vi "CRYMR Min Margin.vi"(3 "Lower X":dbl format="%.2f", 4 "Lower Margin":dbl format="%.2p", 5 "Upper X":dbl format="%.2f", 6 "Upper Margin":dbl format="%.2f") -> (0 "Critical":u16(ring) items=["Upper", "Lower", "Both"], 1 "X":dbl=1.0 format="%.2f", 2 "Min Margin":dbl format="%.2p")   [LabVIEW 2013]
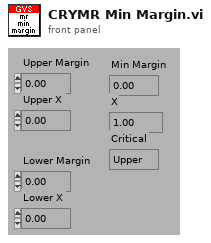
[diagram p1: front panel]
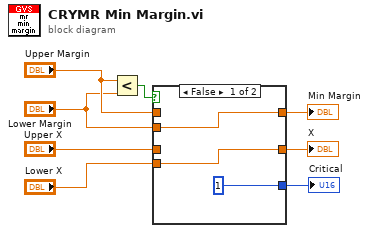
[diagram p0: block diagram]
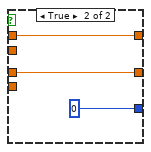
[diagram p2: hidden frame]
diagram:
  n1 = Less?(x="Upper Margin", y="Lower Margin") -> (x < y?=w8:bool)
  n2 = case shown="False" w8 {
    tunnel: "Upper Margin" -> [_ w14]
    tunnel: [w11 w14] -> w6
    tunnel: "Upper X" -> [_ w13]
    tunnel: [w10 w13] -> w4
    tunnel: "Lower Margin" -> [w11 _]
    tunnel: "Lower X" -> [w10 _]
    tunnel: [1 0] -> w1
    frame False {
    }
    frame True {
    }
  }
  "Min Margin" <- w6
  "X" <- w4
  "Critical" <- w1
